vi "GoTo Popup.vi"(2 "error in (no error)":errorcluster, 3 "controller in":refnum<k24>, 4 "axis name":string="X") -> (0 "error out":errorcluster, 1 "controller out":refnum<k24>)   [LabVIEW 2026]
uses:
  <instrlib>/A3200/Bin/Aerotech.A3200.dll
  <instrlib>/A3200/Motion/EnableSingle.vi
  <instrlib>/A3200/Motion/MoveAbsSingle.vi
  <instrlib>/A3200/Motion/AbortSingle.vi
  <instrlib>/A3200/Motion/DisableSingle.vi
panel:
  in  "CANCEL":bool
  in  "Go":bool
  in  "Speed":dbl
  in  "Position":dbl
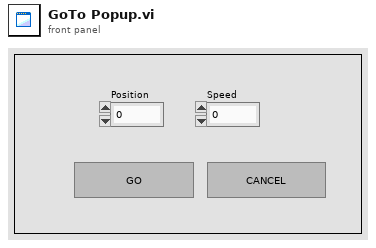
[diagram p1: front panel]
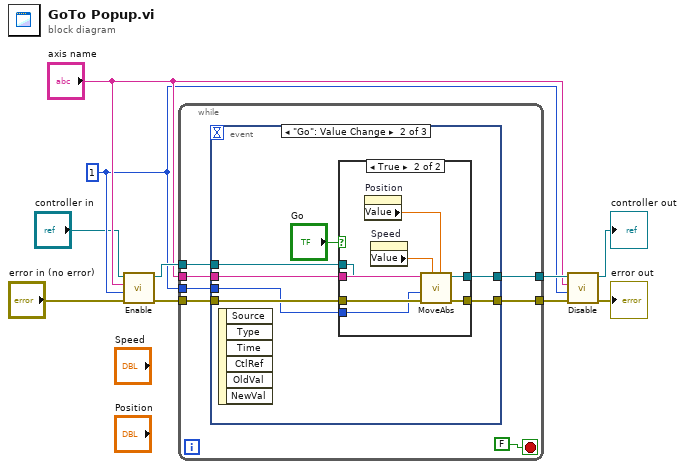
[diagram p0: block diagram]
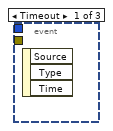
[diagram p2: hidden frame]
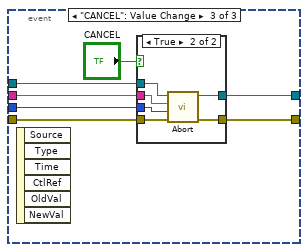
[diagram p4: hidden frame]
diagram:
  w5 = 1 ("taskId")
  n1 = call-poly <instrlib>:"Enable.vi"("error in (no error)"="error in (no error)", "taskId"=w5, "axis name"="axis name", "controller in"="controller in") -> ("error out"=w10:errorcluster, "controller out"=w9:refnum<k24>)  [unwired: 6 in]
  n2 = while {
    tunnel: w9 -> [w17]
    tunnel: w10 -> [w16]
    tunnel: "axis name" -> [w14]
    tunnel: w5 -> [w13]
    tunnel: [w12] -> w8
    tunnel: [w11] -> w7
    stop <- FALSE stop-if-true
    n3 = event shown="[1] \"Go\": Value Change" {
      selector: _ -> [_ _ _]
      dyn-events: _ -> [_ _ _]
      timeout: _ -> [_ _ _]
      tunnel: w17 -> [_ w19 w38]
      tunnel: w16 -> [_ w23 w37]
      tunnel: [_ w22 w36] -> w12
      tunnel: w14 -> [_ w21 w40]
      tunnel: w13 -> [_ w20 w39]
      tunnel: [_ w18 w35] -> w11
      event Timeout {
        n4 = event-data() -> ()  [unwired: 1 in, 3 out]
      }
      event "Go": Value Change {
        n5 = event-data() -> ()  [unwired: 1 in, 6 out]
        n6 = case shown="True" "Go" {
          tunnel: w23 -> [w26 w32]
          tunnel: [w26 w31] -> w22
          tunnel: w21 -> [_ w30]
          tunnel: w20 -> [_ w29]
          tunnel: w19 -> [w25 w28]
          tunnel: [w25 w27] -> w18
          frame False {
          }
          frame True {
            n7 = property on="Position" class="DigNum (strict)"() -> ("Value"=w34:dbl)  [unwired: 2 in, 2 out]
            n8 = property on="Speed" class="DigNum (strict)"() -> ("Value"=w33:dbl)  [unwired: 2 in, 2 out]
            n9 = call-poly <instrlib>:"MoveAbs.vi"("position"=w34, "speed"=w33, "error in (no error)"=w32, "taskId"=w29, "axis name"=w30, "controller in"=w28) -> ("error out"=w31:errorcluster, "controller out"=w27:refnum<k24>)  [unwired: 4 in]
          }
        }
      }
      event "CANCEL": Value Change {
        n10 = event-data() -> ()  [unwired: 1 in, 6 out]
        n11 = case shown="True" "CANCEL" {
          tunnel: w40 -> [_ w49]
          tunnel: w39 -> [_ w48]
          tunnel: w38 -> [w42 w47]
          tunnel: w37 -> [w43 w46]
          tunnel: [w43 w45] -> w36
          tunnel: [w42 w44] -> w35
          frame False {
          }
          frame True {
            n12 = call-poly <instrlib>:"Abort.vi"("error in (no error)"=w46, "taskId"=w48, "axis name? (all)"=w49, "controller in"=w47) -> ("error out"=w45:errorcluster, "controller out"=w44:refnum<k24>)  [unwired: 6 in]
          }
        }
      }
    }
  }
  n13 = call-poly <instrlib>:"Disable.vi"("error in (no error)"=w8, "taskId"=w5, "axis name"="axis name", "controller in"=w7) -> ("error out"=→"error out":errorcluster, "controller out"=→"controller out":refnum<k24>)  [unwired: 6 in]
